vi "createTempControllerBackEndEvents.vi"(8 "error in (no error)":errorcluster, 11 "CameraEventsManger.lvclass in":refnum<class "CameraEventsManger.lvclass">) -> (0 "error out":errorcluster, 2 "tempControllerBackEndEvents":T1, 3 "CameraEventsManger.lvclass out":refnum<class "CameraEventsManger.lvclass">)   [LabVIEW 2009, in "Tools.lvlib" / "Settings.lvlib" / "CameraEventsManger.lvclass"]
uses:
  CameraEventsManger.lvclass
  CameraEventsManger.lvclass/CameraEventsManger.ctl
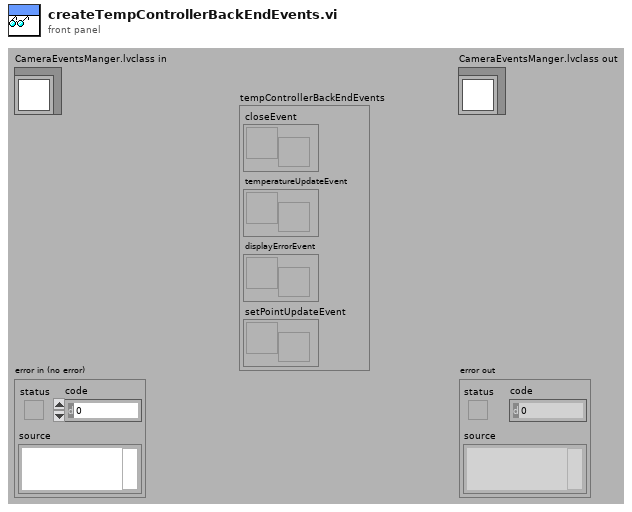
[diagram p1: front panel]
types:
  T1 = cluster{"closeEvent":refnum<user-event>, "temperatureUpdateEvent":refnum<user-event>, "displayErrorEvent":refnum<user-event>, "setPointUpdateEvent":refnum<user-event>}
  T2 = cluster{"closeEvent":cluster{"closeValue":bool}, "temperatureUpdateEvent":cluster{"newTemperature":i32, "Status":string}, "displayErrorEvent":cluster{"errorValue":errorcluster}, "setPointUpdateEvent":cluster{"newTemperature":i32, "CoolerOnOff":bool}}
  T3 = cluster{"newTemperature":i32, "CoolerOnOff":bool}
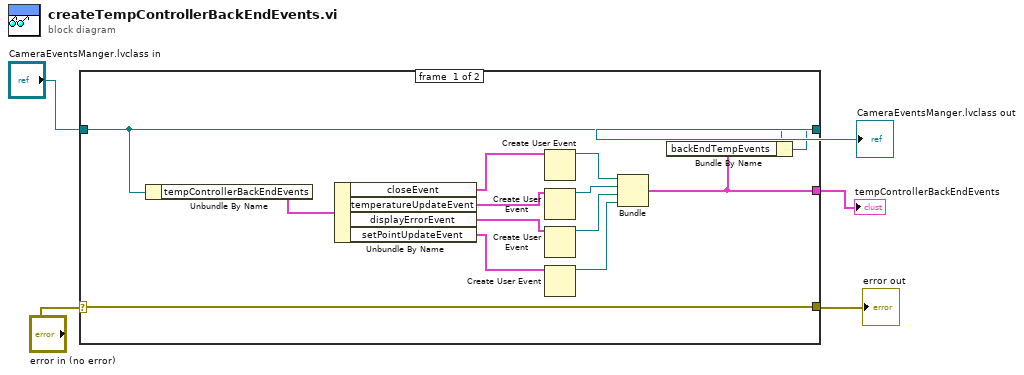
[diagram p0: block diagram]
diagram:
  n1 = case shown="No Error" "error in (no error)" {
    selector: "error in (no error)" -> [w18 w19]
    tunnel: [w18 w19] -> w4
    tunnel: [w6 w20] -> w2
    tunnel: "CameraEventsManger.lvclass in" -> [w7 w20]
    tunnel: [w8 _] -> w1
    frame #0 {
      n2 = Unbundle By Name(w7) -> ("tempControllerBackEndEvents"=w17:T2)
      n3 = Unbundle By Name(w17) -> ("closeEvent"=w16:cluster{"closeValue":bool}, "temperatureUpdateEvent"=w15:cluster{"newTemperature":i32, "Status":string}, "displayErrorEvent"=w14:cluster{"errorValue":errorcluster}, "setPointUpdateEvent"=w13:T3)
      n4 = Create User Event(user event datatype=w16) -> (user event=w12:refnum<user-event>)  [unwired: 1 in, 1 out]
      n5 = Create User Event(user event datatype=w15) -> (user event=w11:refnum<user-event>)  [unwired: 1 in, 1 out]
      n6 = Create User Event(user event datatype=w14) -> (user event=w9:refnum<user-event>)  [unwired: 1 in, 1 out]
      n7 = Create User Event(user event datatype=w13) -> (user event=w10:refnum<user-event>)  [unwired: 1 in, 1 out]
      n8 = Bundle("closeEvent"=w12, "temperatureUpdateEvent"=w11, "displayErrorEvent"=w9, "setPointUpdateEvent"=w10) -> (w8:T1)  [unwired: 1 in]
      n9 = Bundle By Name(cluster=w7, "backEndTempEvents"=w8) -> (w6:refnum<class "CameraEventsManger.lvclass">)
    }
    frame #1 {
    }
  }
  "error out" <- w4
  "CameraEventsManger.lvclass out" <- w2
  "tempControllerBackEndEvents" <- w1
